vi "Init.vi"(11 "Bricks in":refnum<class "Bricks.lvclass">) -> (3 "Bricks out":refnum<class "Bricks.lvclass">)   [LabVIEW 2015, in "Bricks.lvclass"]
uses:
  Bricks.lvclass
  MasonLines.ctl
  Brick Wall Type.ctl
  Type Defs/Direction Enum.ctl
  SpawnLines.ctl
  Bricks.lvclass/Bricks.ctl
  Type Defs/SB Type Defs.lvlib
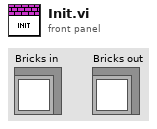
[diagram p1: front panel]
types:
  T1 = typedef "Bricks.lvclass/SpawnLines.ctl" = cluster{"NSpawn":i32, "ESpawn":i32, "SSpawn":i32, "WSpawn":i32}
  T2 = typedef "SB Type Defs.lvlib/Direction Enum.ctl" = enum16{"NW", "N", "NE", "E", "SE", "S", "SW", "W"}
  T3 = typedef "Bricks.lvclass/Brick Wall Type.ctl" = enum16{"Starter", "Spawner", "Mason", "Wall", "Hottie"}
  T4 = typedef "Bricks.lvclass/MasonLines.ctl" = cluster{"NMasonLine":i32, "EMasonLine":i32, "SMasonLine":i32, "WMasonLine":i32}
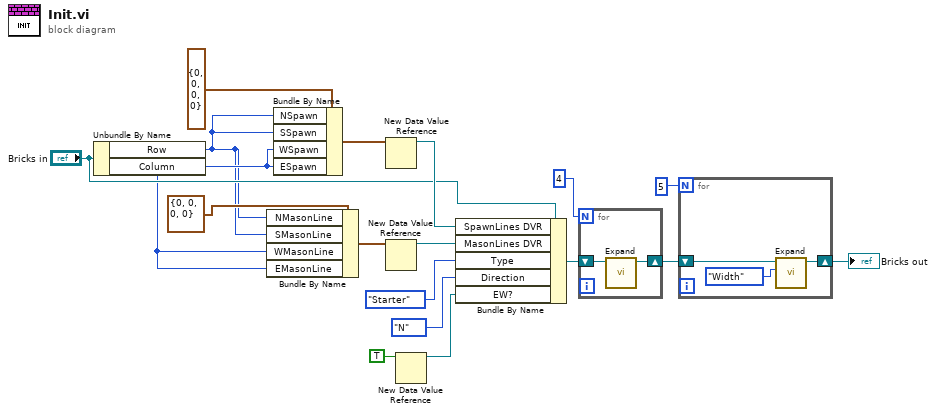
[diagram p0: block diagram]
diagram:
  n1 = Unbundle By Name("Bricks in") -> ("Row"=w1:i32, "Column"=w2:i32)
  n2 = Bundle By Name(cluster=T4 {"NMasonLine"=0, "EMasonLine"=0, "SMasonLine"=0, "WMasonLine"=0} ("MasonLines"), "NMasonLine"=w1, "SMasonLine"=w1, "WMasonLine"=w2, "EMasonLine"=w2) -> (w6:T4)
  n3 = Bundle By Name(cluster=T1 {"NSpawn"=0, "ESpawn"=0, "SSpawn"=0, "WSpawn"=0} ("WallLines"), "NSpawn"=w1, "SSpawn"=w1, "WSpawn"=w2, "ESpawn"=w2) -> (w3:T1)
  n4 = New Data Value Reference(data value=w3) -> (data value reference=w16:refnum<data-value>)  [unwired: 1 in, 1 out]
  n5 = New Data Value Reference(data value=w6) -> (data value reference=w11:refnum<data-value>)  [unwired: 1 in, 1 out]
  n6 = New Data Value Reference(data value=TRUE) -> (data value reference=w18:refnum<data-value>)  [unwired: 1 in, 1 out]
  n7 = Bundle By Name(cluster="Bricks in", "SpawnLines DVR"=w16, "MasonLines DVR"=w11, "Type"=Brick_Wall_Type."Starter" ("Player. Type"), "Direction"=Direction_Enum."N" ("Player.Direction"), "EW?"=w18) -> (w9:refnum<class "Bricks.lvclass">)
  n8 = for {
    N: 4 -> [_]
    shift-right: [w19] -> w7
    shift-left: w9 -> [w20]
    n9 = call-dynamic "Expand.vi"("Brick Wall in"=w20) -> ("Brick Wall out"=w19:refnum<class "Bricks.lvclass">)  [unwired: 9 in, 1 out]
  }
  n10 = for {
    N: 5 -> [_]
    shift-right: [w22] -> w14
    shift-left: w7 -> [w23]
    n11 = call-dynamic "Expand.vi"("Expand Direction"=enum16{"Height", "Width", "Both"}."Width", "Brick Wall in"=w23) -> ("Brick Wall out"=w22:refnum<class "Bricks.lvclass">)  [unwired: 8 in, 1 out]
  }
  "Bricks out" <- w14
